vi "RegisterTrend.vi"(8 "error in":errorcluster, 10 "RegisterTrend":T1, 11 "config":T3) -> (0 "error out":errorcluster, 3 "config":T3)   [LabVIEW 2017, in "IrDataEventCreator.lvlib"]
uses:
  <vilib>/addons/InsightCM/Devices/Shared/Ir/IrDataEventCreator/IrDataEventCreator.lvlib
  <vilib>/addons/InsightCM/Devices/Shared/Ir/IrDataEventCreator/controls/config.ctl
  <vilib>/addons/InsightCM/Devices/Shared/Common/DataEventCreator/controls/RegisterTrendPoints.ctl
  <vilib>/addons/InsightCM/Devices/Shared/Common/DataEventCreator/controls/Registry_Trend.ctl
  <vilib>/addons/InsightCM/Devices/Shared/Ir/IrDataEventCreator/controls/Registry.ctl
  <vilib>/addons/InsightCM/Devices/Shared/Ir/IrDataEventCreator/controls/Registry_Image.ctl
  <vilib>/addons/InsightCM/MessageBus/Base/controls/KeyValuePair.ctl
  <vilib>/addons/InsightCM/Devices/Shared/Common/DataEventCreator/DataEventCreator.lvlib
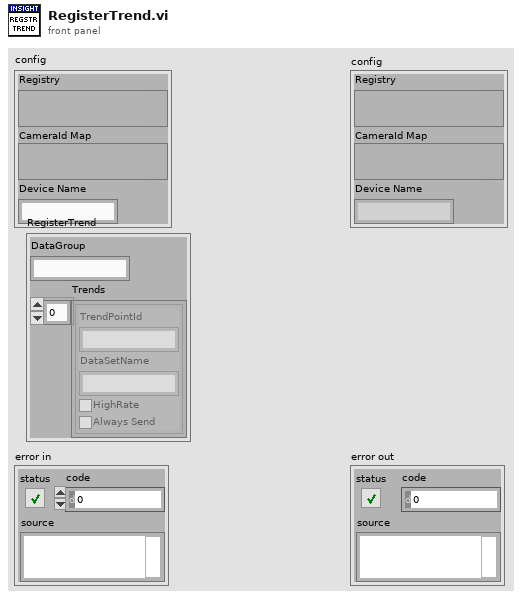
[diagram p1: front panel]
types:
  T1 = typedef "DataEventCreator.lvlib/RegisterTrendPoints.ctl" = cluster{"DataGroup":string, "Trends":T2[]}
  T2 = typedef "DataEventCreator.lvlib/Registry_Trend.ctl" = cluster{"TrendPointId":string, "DataSetName":string, "HighRate":bool, "Always Send":bool}
  T3 = typedef "IrDataEventCreator.lvlib/config.ctl" = cluster{"Registry":variant, "CameraId Map":variant, "Device Name":string}
  T4 = typedef "IrDataEventCreator.lvlib/Registry.ctl" = cluster{"Image":T5, "Trend Points":T2[]}
  T5 = typedef "IrDataEventCreator.lvlib/Registry_Image.ctl" = cluster{"Properties":T6[]}
  T6 = typedef "KeyValuePair.ctl" = cluster{"Key":string, "Value":string}
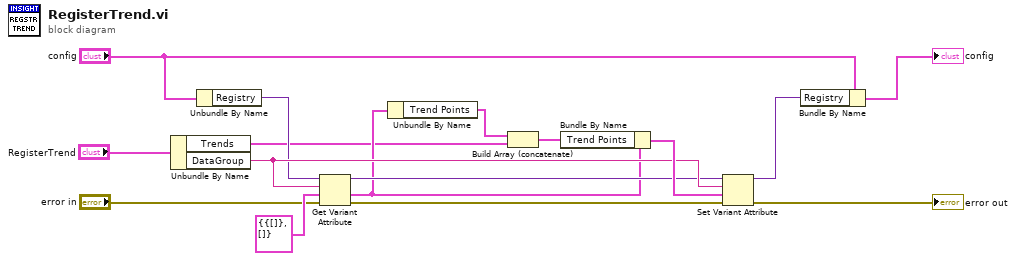
[diagram p0: block diagram]
diagram:
  n1 = Unbundle By Name("RegisterTrend") -> ("Trends"=w3:T2[], "DataGroup"=w11:string)
  n2 = Unbundle By Name("config") -> ("Registry"=w9:variant)
  n3 = Get Variant Attribute(Variant=w9, name=w11, default value (empty Variant)=T4 {"Image"={"Properties"=[]}, "Trend Points"=[]} ("Registry"), error in="error in") -> (duplicate Variant=w10:variant, value=w5:T4, error out=w13:errorcluster)  [unwired: 1 out]
  n4 = Unbundle By Name(w5) -> ("Trend Points"=w4:T2[])
  n5 = Build Array (concatenate)(w4, w3) -> (w2:T2[])
  n6 = Bundle By Name(cluster=w5, "Trend Points"=w2) -> (w12:T4)
  n7 = Set Variant Attribute(Variant=w10, name=w11, value=w12, error in=w13) -> (Variant out=w8:variant, error out=→"error out":errorcluster)  [unwired: 1 out]
  n8 = Bundle By Name(cluster="config", "Registry"=w8) -> (→"config":T3)
